vi "1_Counter_Time_Trace.vi"(8 "error in (no error)":errorcluster) -> (0 "error out":errorcluster)   [LabVIEW 2014]
uses:
  SwabianInstruments.TimeTagger
panel:
  out "XY Graph":cluster{dbl[], "getData":i32[]}[](graph)
  # "The built in test signal (~ 800 to 900 kHz) is applied first to channel 1 and then 1 s later to channel 2."
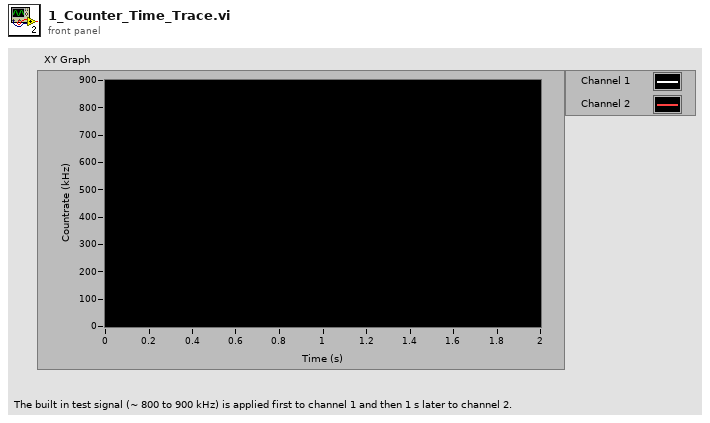
[diagram p1: front panel]
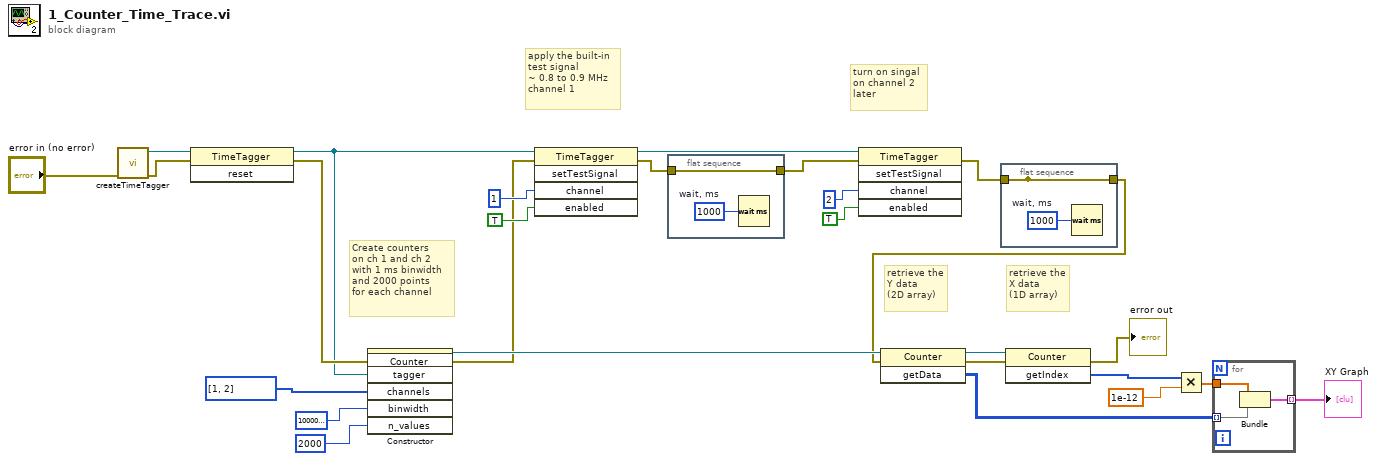
[diagram p0: block diagram]
diagram:
  # "retrieve the\nX data\n(1D array)"
  # "retrieve the\nY data\n(2D array)"
  # "turn on singal\non channel 2\nlater"
  # "apply the built-in\ntest signal\n~ 0.8 to 0.9 MHz\nchannel 1"
  # "Create counters\non ch 1 and ch 2\nwith 1 ms binwidth\nand 2000 points\nfor each channel"
  n1 = call "createTimeTagger.vi"("error in (no error)"="error in (no error)") -> ("error out"=w27:errorcluster, "TimeTagger ref out"=w3:refnum<k24>)  [unwired: 9 in]
  n2 = invoke class="TimeTagger" method="reset"(reference=w3, error in=w27) -> (reference out=w10:refnum<k24>, error out=w26:errorcluster)  [unwired: 1 in, 1 out]
  n3 = constructor class="Counter"(error in=w26, "tagger"=w10, "channels"=i32[] [1, 2], "binwidth"=i64 1000000000, "n_values"=2000) -> (reference out=w25:refnum<k24>, error out=w17:errorcluster)  [unwired: 2 in, 5 out]
  n4 = invoke class="TimeTagger" method="setTestSignal"(reference=w10, error in=w17, "channel"=1, "enabled"=TRUE) -> (reference out=w14:refnum<k24>, error out=w11:errorcluster)  [unwired: 1 in, 3 out]
  n5 = flat-sequence {
    tunnel: [w28] -> w12
    tunnel: w11 -> [w28]
    frame #0 {
      w29 = u32 1000  # wait, ms
      n6 = Wait (ms)(milliseconds to wait=w29) -> ()  [unwired: 1 out]
    }
  }
  n7 = invoke class="TimeTagger" method="setTestSignal"(reference=w14, error in=w12, "channel"=2, "enabled"=TRUE) -> (error out=w5:errorcluster)  [unwired: 1 in, 4 out]
  n8 = invoke class="Counter" method="getData"(reference=w25, error in=w4) -> (reference out=w24:refnum<k24>, error out=w23:errorcluster, "getData"=w8:i32[][])  [unwired: 1 in]
  n9 = flat-sequence {
    tunnel: [w30] -> _
    tunnel: w5 -> [w30]
    tunnel: [w30] -> w4
    frame #0 {
      w31 = u32 1000  # wait, ms
      n10 = Wait (ms)(milliseconds to wait=w31) -> ()  [unwired: 1 out]
    }
  }
  n11 = invoke class="Counter" method="getIndex"(reference=w24, error in=w23) -> (error out=→"error out":errorcluster, "getIndex"=w9:i64[])  [unwired: 1 in, 1 out]
  n12 = Multiply(x=w9, y=1e-12) -> (x*y=w7:dbl[])
  n13 = for {
    tunnel: w8 -> [w33] mode=indexing
    tunnel: w7 -> [w34]
    tunnel: [w32] -> w6 mode=indexing
    n14 = Bundle(w34, "getData"=w33) -> (w32:cluster{dbl[], "getData":i32[]})  [unwired: 1 in]
  }
  "XY Graph" <- w6
